vi "Request and Apply Prefs.vi"(8 "error in (no error)":errorcluster, 11 "GUI Helper in":refnum<class "GUI Helper.lvclass">) -> (0 "error out":errorcluster, 3 "GUI Helper out":refnum<class "GUI Helper.lvclass">)   [LabVIEW 2020, in "VolatusGUI.lvlib" / "GUI Helper.lvclass"]
uses:
  GUI Helper.lvclass
  C:/dev/lv20CE/relink/lv-volatus/Volatus/Module/Module.lvclass
  GUIStateValue/GUIStateValue.lvclass
  GUI Helper.lvclass/GUI Helper.ctl
  Volatus/Module/Module.lvclass/Module.ctl
  Volatus/MessageQ/MessageQ.lvclass
  Volatus/Volatus.lvlib
  Volatus/Module/Module.lvclass
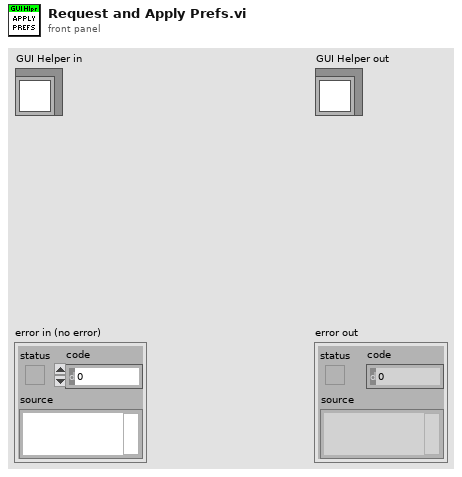
[diagram p1: front panel]
types:
  T1 = typedef "VolatusGUI.lvlib/GUI State.ctl" = cluster{"GUI ID":string, "Visible":bool, "Visibility Set":bool, "Bounds":T2, "Bounds Set":bool}
  T2 = typedef "LVRectTypeDef.ctl" = cluster{"Left":i16, "Top":i16, "Right":i16, "Bottom":i16}
  T3 = typedef "VolatusGUI.lvlib/GUI Helper.lvclass/GUI Properties.ctl" = cluster{"Width":u16, "Height":u16, "Resizable":bool}
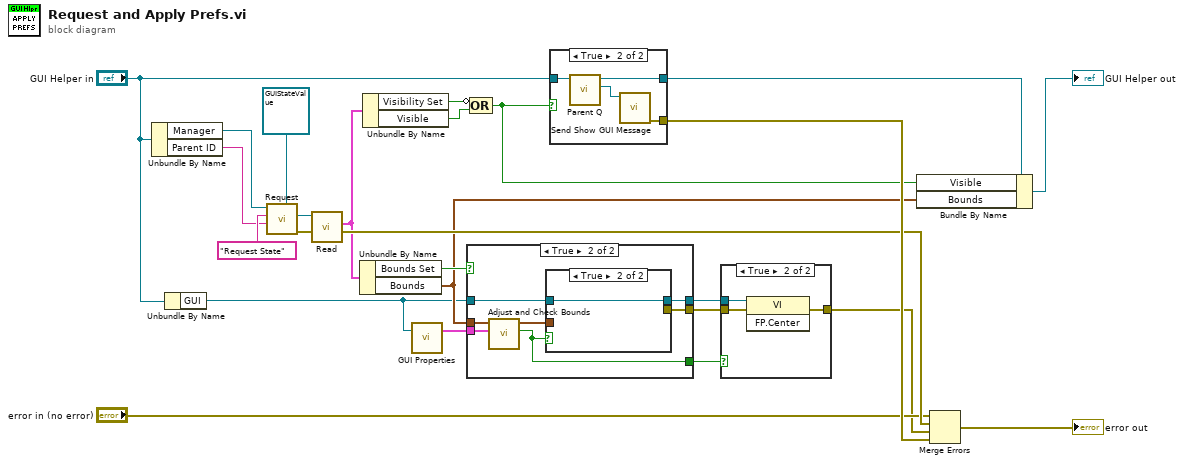
[diagram p0: block diagram]
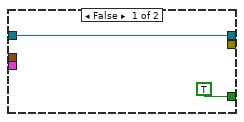
[diagram p4: hidden frame]
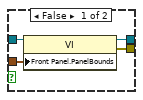
[diagram p5: hidden frame]
diagram:
  n1 = Unbundle By Name("GUI Helper in") -> ("Manager"=w16:refnum<class "MessageQ.lvclass">, "Parent ID"=w1:string)
  n2 = Unbundle By Name("GUI Helper in") -> ("GUI"=w7:refnum<vi>)
  n3 = call "Request.vi"("Response Type (None)"=refnum<class "GUIStateValue.lvclass"> refnum ("VolatusGUI:GUIStateValue.lvclass"), "Data"=w1, "ID"="Request State", "MessageQ in"=w16) -> ("error out"=w23:errorcluster, "Response"=w20:refnum<class "GUIStateValue.lvclass">)  [unwired: 5 in, 1 out]
  n4 = call "Read.vi"("GUIStateValue in"=w20) -> ("GUI State"=w19:T1)  [unwired: 10 in]
  n5 = Unbundle By Name(w19) -> ("Bounds Set"=w18:bool, "Bounds"=w11:T2)
  n6 = Unbundle By Name(w19) -> ("Visibility Set"=w10:bool, "Visible"=w9:bool)
  n7 = call "GUI Properties.vi"("GUI"=w7) -> ("GUI Properties"=w2:T3)  [unwired: 6 in]
  n8 = case shown="True" w18 {
    tunnel: w7 -> [w26 w33]
    tunnel: w11 -> [_ w31]
    tunnel: [_ w32] -> w6
    tunnel: [w26 w27] -> w5
    tunnel: [TRUE w28] -> w3
    tunnel: w2 -> [_ w29]
    frame False {
    }
    frame True {
      n9 = call "Adjust and Check Bounds.vi"("GUI Properties"=w29, "Saved Bounds"=w31) -> ("Center"=w28:bool, "Bounds"=w30:T2)  [unwired: 8 in]
      n10 = case shown="True" w28 {
        tunnel: w33 -> [w37 w38]
        tunnel: [w36 _] -> w32
        tunnel: w30 -> [w35 _]
        tunnel: [w34 w38] -> w27
        frame False {
          n11 = property class="VI"(reference=w37, "Front Panel.PanelBounds"=w35) -> (reference out=w34:refnum<vi>, error out=w36:errorcluster)  [unwired: 1 in]
        }
        frame True {
        }
      }
    }
  }
  n12 = Compound Arithmetic op=OR(invert w10, w9) -> (w8:bool)
  n13 = case shown="True" w8 {
    tunnel: "GUI Helper in" -> [w39 w43]
    tunnel: [w39 w41] -> w15
    tunnel: [_ w40] -> w24
    frame False {
    }
    frame True {
      n14 = call "Parent Q.vi"("Module in"=w43) -> ("Parent Q"=w42:refnum<class "MessageQ.lvclass">, "Module out"=w41:refnum<class "GUI Helper.lvclass">)  [unwired: 9 in]
      n15 = call "Send Show GUI Message.vi"("MessageQ"=w42) -> ("error out"=w40:errorcluster)  [unwired: 10 in]
    }
  }
  n16 = case shown="True" w3 {
    tunnel: w6 -> [w44 w47]
    tunnel: w5 -> [_ w46]
    tunnel: [w44 w45] -> w4
    frame False {
    }
    frame True {
      n17 = invoke class="VI" method="FP.Center"(reference=w46, error in=w47) -> (error out=w45:errorcluster)  [unwired: 1 in, 2 out]
    }
  }
  n18 = Bundle By Name(cluster=w15, "Visible"=w8, "Bounds"=w11) -> (→"GUI Helper out":refnum<class "GUI Helper.lvclass">)
  n19 = Merge Errors("error in (no error)", w23, w4, w24) -> (→"error out":errorcluster)
